vi "matchedFilterKernel.vi"(9 "theta":dbl, 10 "sigma":dbl, 11 "L":dbl) -> (3 "Array":dbl[][](array[numeric]))   [LabVIEW 2020]
uses:
  <vilib>/Analysis/coordinate.llb/2D Cartesian Coordinate Rotation (Array).vi
  <vilib>/Analysis/NI_AALPro.lvlib
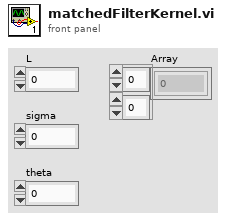
[diagram p1: front panel]
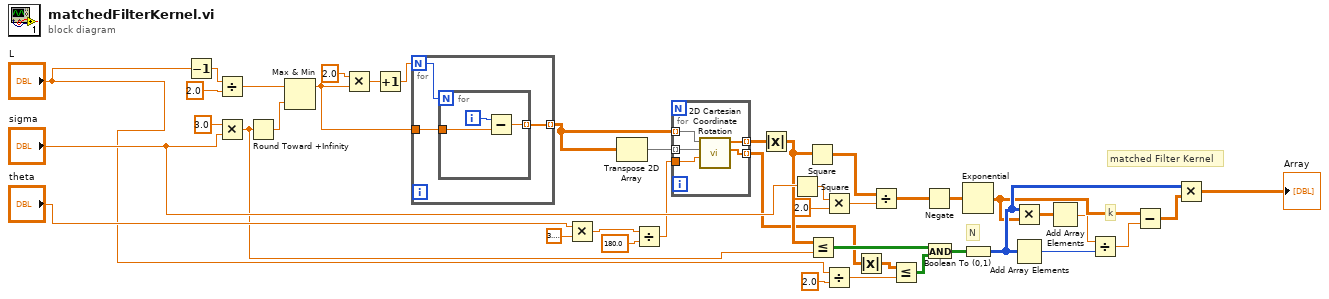
[diagram p0: block diagram]
diagram:
  # "matched Filter Kernel"
  # "k"
  # "N"
  n1 = Decrement(x="L") -> (x-1=w2:dbl)
  n2 = Divide(x=w2, y=2.0) -> (x/y=w4:dbl)
  n3 = Multiply(x=3.0, y="sigma") -> (x*y=w17:dbl)
  n4 = Round Toward +Infinity(x=w17) -> (ceil(x): smallest int >= x=w5:dbl)
  n5 = Max & Min(x=w4, y=w5) -> (max(x,y)=w7:dbl)  [unwired: 1 out]
  n6 = Multiply(x=2.0, y=w7) -> (x*y=w8:dbl)
  n7 = Increment(x=w8) -> (x+1=w9:dbl)
  n8 = for {
    N: w9 -> [w43]
    tunnel: w7 -> [w45]
    tunnel: [w44] -> w10 mode=indexing
    n9 = for {
      N: w43 -> [_]
      tunnel: w45 -> [w47]
      tunnel: [w46] -> w44 mode=indexing
      i -> [w48]
      n10 = Subtract(x=w48, y=w47) -> (x-y=w46:dbl)
    }
  }
  n11 = Multiply(x="theta", y=3.141592653589793) -> (x*y=w13:dbl)
  n12 = Transpose 2D Array(2D array=w10) -> (transposed array=w11:dbl[][])
  n13 = Divide(x=w13, y=180.0) -> (x/y=w15:dbl)
  n14 = for {
    tunnel: w10 -> [w53] mode=indexing
    tunnel: w11 -> [w52] mode=indexing
    tunnel: [w51] -> w16 mode=indexing
    tunnel: [w50] -> w19 mode=indexing
    tunnel: w15 -> [w49]
    n15 = call-poly <vilib>:"2D Cartesian Coordinate Rotation.vi"("theta"=w49, "Y"=w52, "X"=w53) -> ("Y Out"=w50:dbl[], "X Out"=w51:dbl[])  [unwired: 6 in, 1 out]
  }
  n16 = Absolute Value(x=w16) -> (abs(x)=w30:dbl[][])
  n17 = Square(x="sigma") -> (x^2=w28:dbl)
  n18 = Square(x=w30) -> (x^2=w31:dbl[][])
  n19 = Less Or Equal?(x=w30, y=w17) -> (x <= y?=w23:bool[][])
  n20 = Multiply(x=w28, y=2.0) -> (x*y=w27:dbl)
  n21 = Divide(x="L", y=2.0) -> (x/y=w22:dbl)
  n22 = Absolute Value(x=w19) -> (abs(x)=w18:dbl[][])
  n23 = Divide(x=w31, y=w27) -> (x/y=w26:dbl[][])
  n24 = Less Or Equal?(x=w18, y=w22) -> (x <= y?=w24:bool[][])
  n25 = Negate(x=w26) -> (-x=w25:dbl[][])
  n26 = And(x=w23, y=w24) -> (x .and. y?=w33:bool[][])
  n27 = Exponential(1:w25) -> (0:w37:dbl[][])
  n28 = Boolean To (0,1)(Boolean=w33) -> (0, 1=w39:i16[][])
  n29 = Multiply(x=w39, y=w37) -> (x*y=w34:dbl[][])
  n30 = Add Array Elements(numeric array=w39) -> (sum=w36:i16)
  n31 = Add Array Elements(numeric array=w34) -> (sum=w35:dbl)
  n32 = Divide(x=w35, y=w36) -> (x/y=w38:dbl)
  n33 = Subtract(x=w37, y=w38) -> (x-y=w40:dbl[][])
  n34 = Multiply(x=w39, y=w40) -> (x*y=→"Array":dbl[][])
